vi "okCFrontPanel Set Wire In Value.vi"(8 "Error In":errorcluster, 9 "Value":u32, 10 "Endpoint":i32, 11 "okCFrontPanel Refnum":refnum<k24>) -> (0 "Error Out":errorcluster, 3 "okCFrontPanel Refnum":refnum<k24>)   [LabVIEW 2019, in "okFrontPanelC#Wrapper.lvlib"]
uses:
  okFrontPanelC#Wrapper.lvlib
  C:/UCLA Thinkpad Google Drive/LabVIEW 2019 SP1/builds/SS2 Live Distribution/Opal Kelly/C# Wrapper/libFrontPanel-csharp.dll
  libFrontPanel-csharp.dll
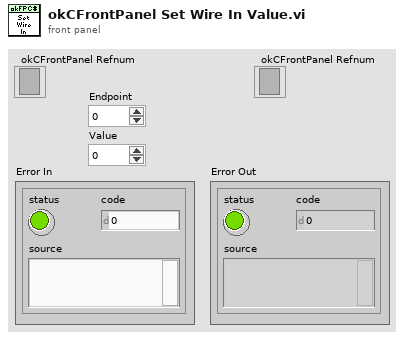
[diagram p1: front panel]
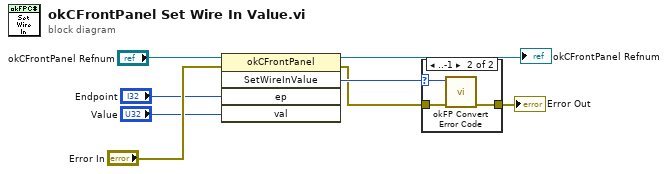
[diagram p0: block diagram]
diagram:
  n1 = invoke class="okCFrontPanel" method="SetWireInValue"(reference="okCFrontPanel Refnum", error in="Error In", "ep"="Endpoint", "val"="Value") -> (reference out=→"okCFrontPanel Refnum":refnum<k24>, error out=w4:errorcluster, "SetWireInValue"=w5:i32)  [unwired: 1 in, 2 out]
  n2 = case shown="..-1" w5 {
    selector: w5 -> [_ w12]
    tunnel: w4 -> [w9 w11]
    tunnel: [w9 w10] -> w3
    frame 0, Default {
    }
    frame ..-1 {
      n3 = call "okFP Convert Error Code.vi"("error in (no error)"=w11, "okFP Error Code"=w12) -> ("error out"=w10:errorcluster)  [unwired: 9 in]
    }
  }
  "Error Out" <- w3
